vi "Set NI-DAQ Output.vi"(4 "State":bool, 6 "Channel":refnum<k21>="Vacuum", 8 "error in (no error)":errorcluster) -> (0 "error out":errorcluster)   [LabVIEW 2015]
uses:
  <vilib>/DAQmx/write.llb/DAQmx Write (Digital Bool 1Line 1Point).vi
  <vilib>/DAQmx/miscellaneous.llb/DAQmx Fill In Error Info.vi
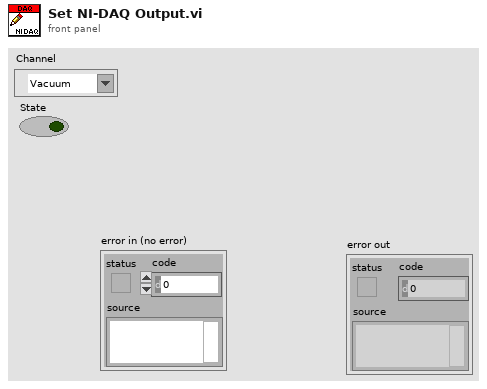
[diagram p1: front panel]
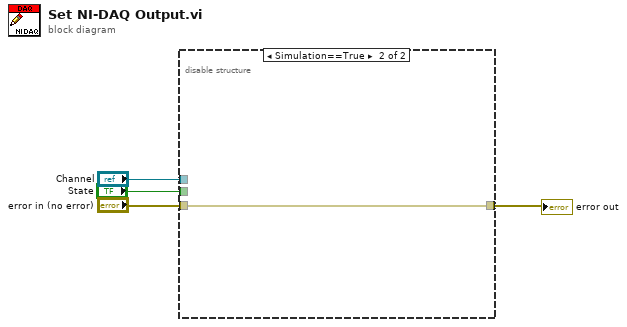
[diagram p0: block diagram]
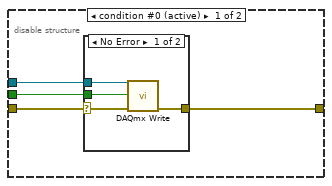
[diagram p2: hidden frame]
diagram:
  n1 = disable-structure shown="Simulation==True" {
    disable-tunnel: [w8 w14] -> w4
    disable-tunnel: "error in (no error)" -> [w7 w14]
    disable-tunnel: "Channel" -> [w6 _]
    disable-tunnel: "State" -> [w5 _]
    frame condition #0 (active) {
      n2 = case shown="No Error" w7 {
        selector: w7 -> [w11 w13]
        tunnel: [w9 w13] -> w8
        tunnel: w6 -> [w12 _]
        tunnel: w5 -> [w10 _]
        frame No Error {
          n3 = call-poly <vilib>:"DAQmx Write.vi"("task/channels in"=w12, "data"=w10, "error in"=w11) -> ("error out"=w9:errorcluster)  [unwired: 10 in, 2 out]
        }
        frame Error {
        }
      }
    }
    frame condition #1 {
    }
  }
  "error out" <- w4
